vi "Remove Ports Section.vi"(8 "error in":errorcluster, 11 "custom device ref":T1 format="%.0x") -> (0 "error out":errorcluster, 3 "custom device ref out":T1 format="%.0x")   [LabVIEW 2020, in "AIM ARINC 429 Scripting.lvlib"]
uses:
  AIM ARINC 429 Scripting.lvlib
  <vilib>/NI VeriStand/Custom Device API/Custom Device Item Ref.ctl
  Constants.vi
  <vilib>/NI VeriStand/Custom Device Tools/Custom Device Utility Library/NI VeriStand - Search for Item by GUID.vi
  <vilib>/NI VeriStand/Custom Device API/Custom Device API.lvlib
  <vilib>/NI VeriStand/Custom Device Tools/Custom Device Utility Library/Custom Device Utility Library.lvlib
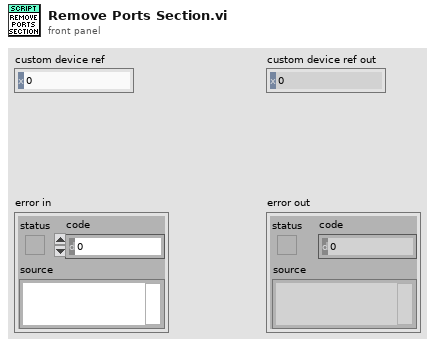
[diagram p1: front panel]
types:
  T1 = typedef "Custom Device API.lvlib/Custom Device Item Ref.ctl" = u64
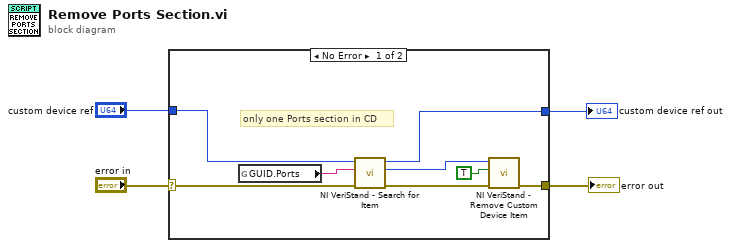
[diagram p0: block diagram]
diagram:
  n1 = case shown="No Error" "error in" {
    selector: "error in" -> [w10 w14]
    tunnel: [w11 w14] -> w4
    tunnel: "custom device ref" -> [w8 w13]
    tunnel: [w5 w13] -> w1
    frame No Error {
      # "only one Ports section in CD"
      n2 = global read "Constants.vi" "GUID.Ports"() -> (w7:string)
      n3 = call-poly <vilib>:"NI VeriStand - Search for Item.vi"("error in"=w10, "Item GUID"=w7, "Section Ref in"=w8) -> ("error out"=w9:errorcluster, "Item Ref"=w6:T1, "Section Ref out"=w5:T1)  [unwired: 5 in, 1 out]
      n4 = call <vilib>:"NI VeriStand - Remove Custom Device Item.vi"("error in (no error)"=w9, "Force Delete (F)"=TRUE, "Item Ref in"=w6) -> ("error out"=w11:errorcluster)  [unwired: 7 in, 1 out]
    }
    frame Error {
    }
  }
  "error out" <- w4
  "custom device ref out" <- w1
